vi "Focus_calc_steps.vi"(9 "Motor steps #":i32=24, 10 "Move (mm)":dbl) -> (1 "Travel (mm)  for motor steps #":dbl format="%#.3g", 2 "#  motor steps for Move (mm)":i32)   [LabVIEW 2021]
panel:
  out "Motor steps per mm":dbl=3936.0
  out "Move position error (mm)":dbl format="%#.3g"
  out "Travel  (mm)  per lead screw turns":dbl
  out "Steps per lead screw turns":i32=3936
  in  "Number of turns reducer/lead screw":dbl=1.0
  in  "Drive stage config":T1={"Motor steps/turn"=24.0, "Microstepping"=1.0, "Lead screw pitch"=20.0, "Gear Ratio "=41} {"Lead screw pitch" min=1.0; "Motor steps/turn" min=1.0}
  out "Travel per motor step (mm)":dbl=3936.0
  out "Travel per lead screw/reducer turn  (mm)":dbl
  out "Motor steps per reducer/lead screw turn":dbl=3936.0
  # "YJ stage: \n\nM01-R1000:100:100 - \n\nmotor 0 is YJ focusing stage: \nnegative is towards the motor \ntotal number of steps to travel ~ 8600 \n\nHK stage: \n\nM11-R1000:100:100\nmotor 1 is HK focusing stage: \nnegative is towards the motor \ntotal number of steps to travel ~ 8600\n\n1 turn of the lead screw is  984 steps  \n\nLead screws thread is 1/24 \" = \n1.058 mm/reducer shaft turn"
  # "Defualt values RATIR(?): \nBoard 1 \ngear ratio : 41\nScrew pitch:  28\nWorm pitch : 1\nMicrosteps: 10\nMotor steps per turn: 24\n\nturns/mm: 45.1969\nsteps/mm: 10847.24\nsteps/inch: 275520.00"
  # "New dafault config 2019: ead screw chanbegd to 1/4-20 \nGear ratio 41 \nLead screw pitch 20 \nMotor steps/turn 24 (15 deg / step)\nmicrostepping 1 \n\nprevious config : \nGear ratio 41 \nLead screw pitch 24 \nMotor steps/turn 24 (15 deg / step)\nmicrostepping 1"
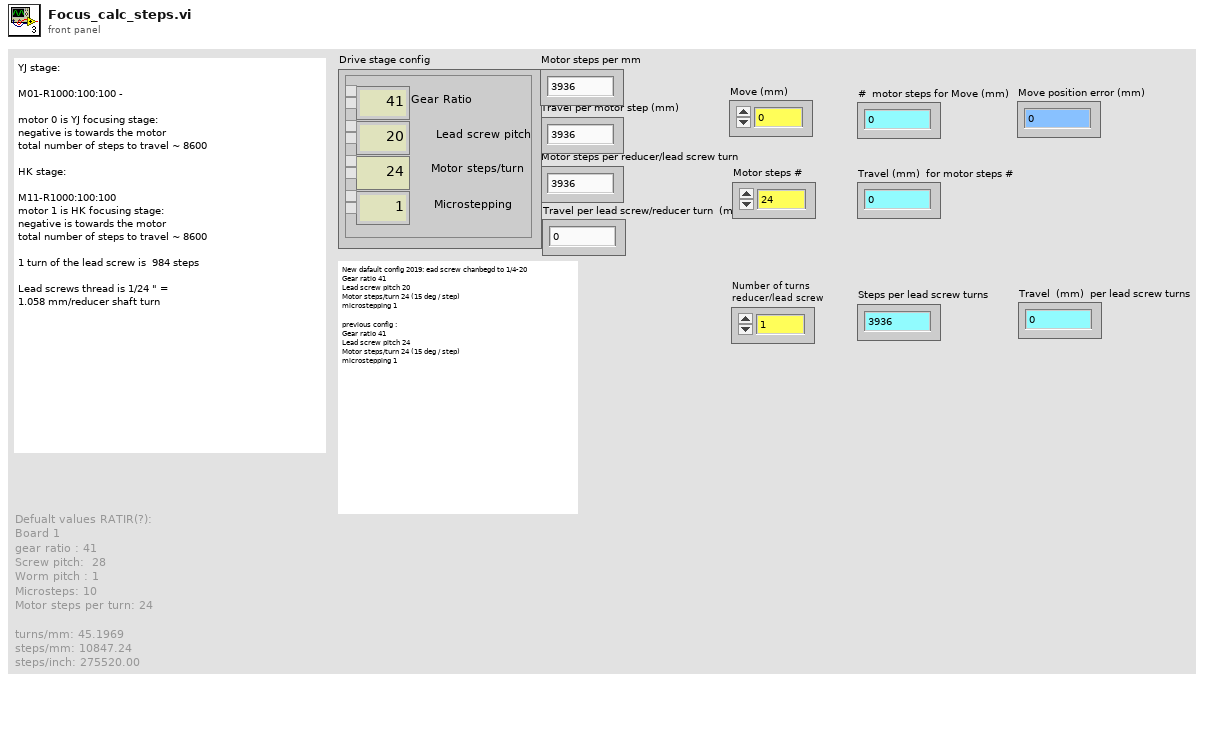
[diagram p1: front panel]
types:
  T1 = cluster{"Motor steps/turn":dbl, "Microstepping":dbl, "Lead screw pitch":dbl, "Gear Ratio ":u16}
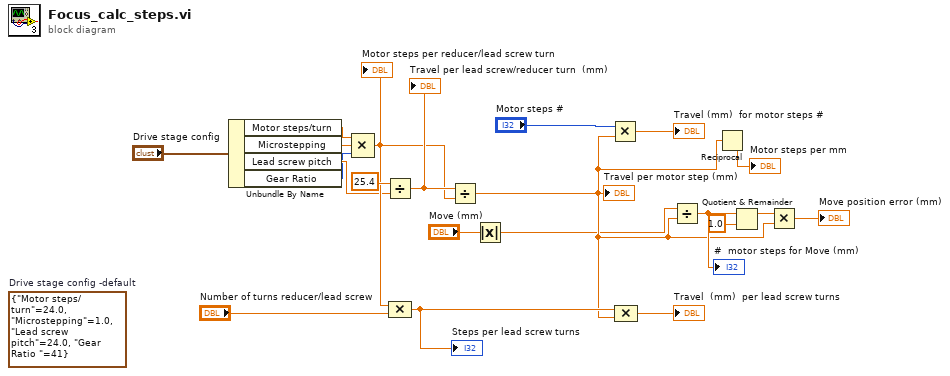
[diagram p0: block diagram]
diagram:
  (unwired) T1 {"Motor steps/turn"=24.0, "Microstepping"=1.0, "Lead screw pitch"=24.0, "Gear Ratio "=41}  # Drive stage config -default
  n1 = Unbundle By Name("Drive stage config") -> ("Motor steps/turn"=w8:dbl, "Microstepping"=w7:dbl, "Lead screw pitch"=w9:dbl, "Gear Ratio"=w6:u16)
  n2 = Compound Arithmetic op=MULTIPLY(w8, w7, w6) -> (w16:dbl)
  "Motor steps per reducer/lead screw turn" <- w16
  n3 = Divide(x=25.4, y=w9) -> (x/y=w19:dbl)
  "Travel per lead screw/reducer turn  (mm)" <- w19
  n4 = Compound Arithmetic op=MULTIPLY(w16, "Number of turns reducer/lead screw") -> (w17:dbl)
  "Steps per lead screw turns" <- w17
  n5 = Divide(x=w19, y=w16) -> (x/y=w2:dbl)
  "Travel per motor step (mm)" <- w2
  n6 = Absolute Value(x="Move (mm)") -> (abs(x)=w1:dbl)
  n7 = Multiply(x="Motor steps #", y=w2) -> (x*y=→"Travel (mm)  for motor steps #":dbl)
  n8 = Compound Arithmetic op=MULTIPLY(w17, w2) -> (→"Travel  (mm)  per lead screw turns":dbl)
  n9 = Divide(x=w1, y=w2) -> (x/y=w13:dbl)
  "#  motor steps for Move (mm)" <- w13
  n10 = Reciprocal(x=w2) -> (1/x=→"Motor steps per mm":dbl)
  n11 = Quotient & Remainder(x=w13, y=1.0) -> (x-y*floor(x/y)=w11:dbl)  [unwired: 1 out]
  n12 = Multiply(x=w11, y=w2) -> (x*y=→"Move position error (mm)":dbl)
